vi "Agilent VNA Set Trace Status.vi"(4 "Trace":i8=1 min=1 max=99 step=1, 6 "Channel":i8=1 min=1 max=99 step=1, 7 "Agilent VNA":T1, 8 "error in (no error)":errorcluster, 10 "Measurements":string[](array[string]), 11 "VISA Resource Name":refnum<visa-resource-name>) -> (0 "error out":errorcluster, 3 "dup VISA Resource Name":refnum<visa-resource-name>)   [LabVIEW 2011]
uses:
  TypeDefs/Agilent VNA Instrument Info.ctl
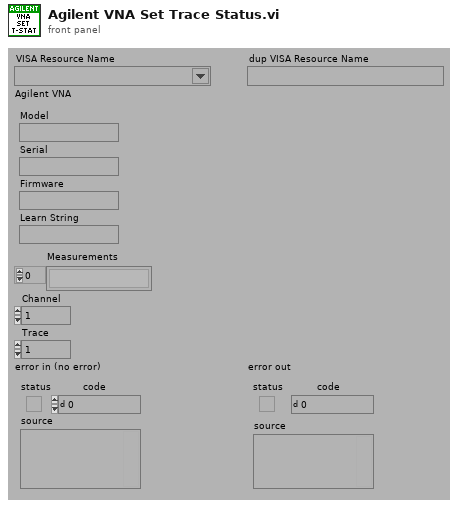
[diagram p1: front panel]
types:
  T1 = typedef "Agilent VNA Instrument Info.ctl" = cluster{"Model":string, "Serial":string, "Firmware":string, "Learn String":string}
  T2 = typedef "Agilent VNA Model.ctl" = enum16{"Not Supported", "8510X", "8719X", "8720X", "8722X", "8753X", "ENA", "PNA", "Field Fox"}
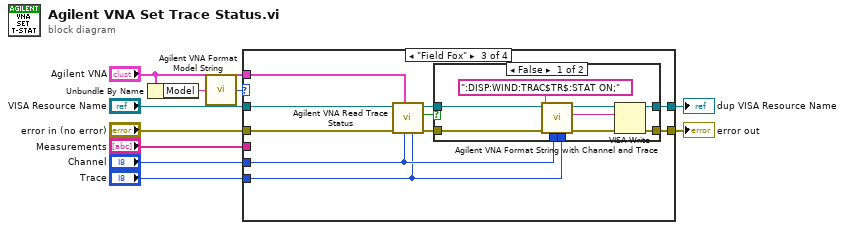
[diagram p0: block diagram]
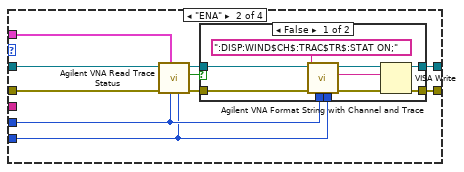
[diagram p3: hidden frame]
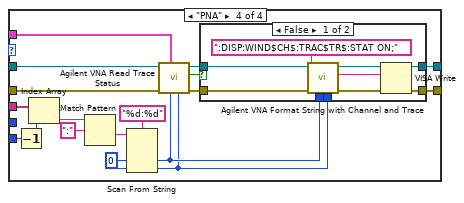
[diagram p6: hidden frame]
diagram:
  n1 = Unbundle By Name("Agilent VNA") -> ("Model"=w3:string)
  n2 = call "Agilent VNA Format Model String.vi"("Model"=w3) -> ("Model"=w6:T2)
  n3 = case shown="\"Field Fox\"" w6 {
    tunnel: "VISA Resource Name" -> [w12 w19 w39 w67]
    tunnel: "error in (no error)" -> [w11 w20 w40 w68]
    tunnel: [w12 w22 w42 w70] -> w8
    tunnel: [w11 w21 w41 w69] -> w7
    tunnel: "Channel" -> [_ w15 w35 _]
    tunnel: "Agilent VNA" -> [_ w16 w36 w64]
    tunnel: "Trace" -> [_ w14 w34 w58]
    tunnel: "Measurements" -> [_ _ _ w62]
    frame "Not Supported".."8753X" {
    }
    frame "ENA" {
      n4 = call "Agilent VNA Read Trace Status.vi"("Trace"=w14, "Channel"=w15, "Agilent VNA"=w16, "error in (no error)"=w20, "VISA Resource Name"=w19) -> ("error out"=w17:errorcluster, "On?"=w13:bool, "dup VISA Resource Name"=w18:refnum<visa-resource-name>)  [unwired: 4 out]
      n5 = case shown="False" w13 {
        tunnel: [w30 w32] -> w22
        tunnel: [w29 w31] -> w21
        tunnel: w18 -> [w28 w32]
        tunnel: w17 -> [w27 w31]
        tunnel: w15 -> [w24 _]
        tunnel: w14 -> [w23 _]
        frame False {
          n6 = call "Agilent VNA Format String with Channel and Trace.vi"("Trace"=w23, "Channel"=w24, "String"=":DISP:WIND$CH$:TRAC$TR$:STAT ON;" ("write buffer")) -> ("String Out"=w26:string)  [unwired: 6 out]
          n7 = VISA Write(VISA resource name=w28, write buffer=w26, error in (no error)=w27) -> (VISA resource name out=w30:refnum<visa-resource-name>, error out=w29:errorcluster)  [unwired: 1 out]
        }
        frame True {
        }
      }
    }
    frame "Field Fox" {
      n8 = call "Agilent VNA Read Trace Status.vi"("Trace"=w34, "Channel"=w35, "Agilent VNA"=w36, "error in (no error)"=w40, "VISA Resource Name"=w39) -> ("error out"=w37:errorcluster, "On?"=w33:bool, "dup VISA Resource Name"=w38:refnum<visa-resource-name>)  [unwired: 4 out]
      n9 = case shown="False" w33 {
        tunnel: [w50 w52] -> w42
        tunnel: [w49 w51] -> w41
        tunnel: w38 -> [w48 w52]
        tunnel: w37 -> [w47 w51]
        tunnel: w35 -> [w44 _]
        tunnel: w34 -> [w43 _]
        frame False {
          n10 = call "Agilent VNA Format String with Channel and Trace.vi"("Trace"=w43, "Channel"=w44, "String"=":DISP:WIND:TRAC$TR$:STAT ON;" ("write buffer")) -> ("String Out"=w46:string)  [unwired: 6 out]
          n11 = VISA Write(VISA resource name=w48, write buffer=w46, error in (no error)=w47) -> (VISA resource name out=w50:refnum<visa-resource-name>, error out=w49:errorcluster)  [unwired: 1 out]
        }
        frame True {
        }
      }
    }
    frame "PNA" {
      w53 = i8 0 ("default value 1")
      n12 = Decrement(x=w58) -> (x-1=w61:i8)
      n13 = Index Array(array=w62, index=w61) -> (element=w55:string)
      n14 = Match Pattern(string=w55, regular expression=":") -> (after substring=w54:string)  [unwired: 1 in, 3 out]
      n15 = Scan From String(format string="%d:%d", input string=w54, default 1=w53, default 2=w53) -> (output 1=w59:i8, output 2=w57:i8)  [unwired: 2 in, 3 out]
      n16 = call "Agilent VNA Read Trace Status.vi"("Trace"=w57, "Channel"=w59, "Agilent VNA"=w64, "error in (no error)"=w68, "VISA Resource Name"=w67) -> ("error out"=w65:errorcluster, "On?"=w63:bool, "dup VISA Resource Name"=w66:refnum<visa-resource-name>)  [unwired: 4 out]
      n17 = case shown="False" w63 {
        tunnel: [w78 w80] -> w70
        tunnel: [w77 w79] -> w69
        tunnel: w66 -> [w76 w80]
        tunnel: w65 -> [w75 w79]
        tunnel: w59 -> [w72 _]
        tunnel: w57 -> [w71 _]
        frame False {
          n18 = call "Agilent VNA Format String with Channel and Trace.vi"("Trace"=w71, "Channel"=w72, "String"=":DISP:WIND$CH$:TRAC$TR$:STAT ON;" ("write buffer")) -> ("String Out"=w74:string)  [unwired: 6 out]
          n19 = VISA Write(VISA resource name=w76, write buffer=w74, error in (no error)=w75) -> (VISA resource name out=w78:refnum<visa-resource-name>, error out=w77:errorcluster)  [unwired: 1 out]
        }
        frame True {
        }
      }
    }
  }
  "dup VISA Resource Name" <- w8
  "error out" <- w7
